vi "XML Parse DBL Liste.vi"(3 "Attribut Name":string, 7 "XML Response":string, 8 "Anzahl Elemente":i32) -> (0 "Background Daten":cluster{"Ramp Pattern":dbl[], dbl[]}[](array[cluster]), 2 "XML Response gekürzt":string)   [LabVIEW 2020, in "FT-IR.lvlib" / "TOOLweb Interface.lvlib" / "TOOLweb Interface Hilfs-VIs.lvlib"]
doc: "Sucht in dem XML-Poll-Response-String \"XML-Response\" den Eintrag mit dem Elementnamen \"Attribut Name\" und liefert dessen Werte im DBL-Array \"Werte\". \n\nDer Eintrag wird dann entfernt, damit eine weiteres Parser-VI am Ausgang \"XML Response gekürzt\" nicht wieder den ganzen String durchsuchen muss."
uses:
  TOOLweb Interface Hilfs-VIs.lvlib
  <vilib>/Analysis/1siggen.llb/Ramp Pattern by Samples.vi
  <vilib>/Analysis/NI_AALBase.lvlib
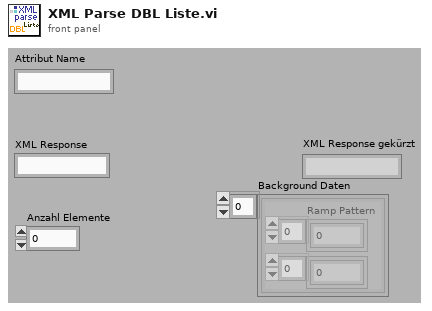
[diagram p1: front panel]
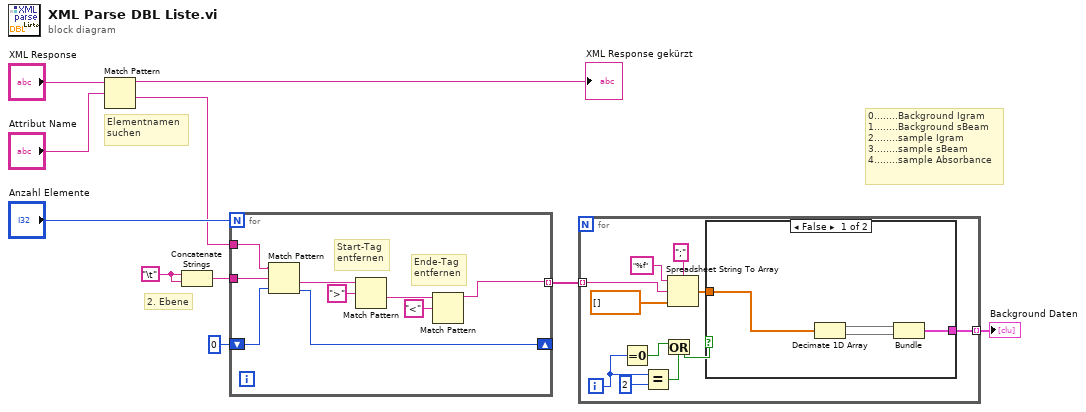
[diagram p0: block diagram]
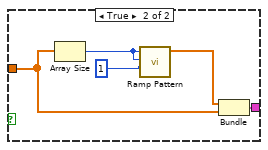
[diagram p2: hidden frame]
diagram:
  w7 = "\t"
  # "0........Background Igram\n1........Background sBeam\n2........sample Igram\n3........sample sBeam\n4........sample Absorbance"
  # "2. Ebene"
  # "Elementnamen\nsuchen"
  n1 = Match Pattern(string="XML Response", regular expression="Attribut Name") -> (before substring=→"XML Response gekürzt":string, after substring=w3:string)  [unwired: 3 out]
  n2 = Concatenate Strings(w7, w7) -> (w6:string)
  n3 = for {
    N: "Anzahl Elemente" -> [_]
    tunnel: w3 -> [w19]
    tunnel: w6 -> [w18]
    shift-right: [w16] -> _
    shift-left: 0 ("offset past match") -> [w17]
    tunnel: [w11] -> w2 mode=indexing
    # "Start-Tag\nentfernen"
    # "Ende-Tag\nentfernen"
    n4 = Match Pattern(string=w19, regular expression=w18, offset (0)=w17) -> (after substring=w15:string, offset past match=w16:i32)  [unwired: 2 out]
    n5 = Match Pattern(string=w15, regular expression=">" ("Regulärer Ausdruck")) -> (after substring=w12:string)  [unwired: 4 out]
    n6 = Match Pattern(string=w12, regular expression="<" ("Regulärer Ausdruck")) -> (before substring=w11:string)  [unwired: 4 out]
  }
  n7 = for {
    tunnel: w2 -> [w28] mode=indexing
    tunnel: [w20] -> w1 mode=indexing
    i -> [w26]
    n8 = Equal To 0?(x=w26) -> (x = 0?=w24:bool)
    n9 = Equal?(x=w26, y=2) -> (x = y?=w23:bool)
    n10 = Or(x=w24, y=w23) -> (x .or. y?=w22:bool)
    n11 = Spreadsheet String To Array(delimiter (Tab)=";", format string="%f", spreadsheet string=w28, array type (2D Dbl)=dbl[] []) -> (array=w21:dbl[])
    n12 = case shown="False" w22 {
      tunnel: w21 -> [w34 w39]
      tunnel: [w31 w35] -> w20
      frame False {
        n13 = Decimate 1D Array(w34) -> (w33:dbl[], w32:dbl[])
        n14 = Bundle(w33, w32) -> (w31:cluster{dbl[], dbl[]})  [unwired: 1 in]
      }
      frame True {
        n15 = Array Size(array=w39) -> (size(s)=w38:i32)
        n16 = call-poly <vilib>:"Ramp Pattern.vi"("start"=1 ("Größe(n)"), "end"=w38, "samples"=w38) -> ("Ramp Pattern"=w36:dbl[])  [unwired: 7 in, 1 out]
        n17 = Bundle("Ramp Pattern"=w36, w39) -> (w35:cluster{"Ramp Pattern":dbl[], dbl[]})  [unwired: 1 in]
      }
    }
  }
  "Background Daten" <- w1
